vi "HEWH Set Draw Condition.vi"(6 "Station":string, 7 "Condition":T1, 8 "Error In":errorcluster, 9 "Station A Test Sequence":T2[](array[typedef])=[{"Sequence #"=0.0, "Cycles"=0, "Mode Setting"="", "Flow Rate (GPM)"=0.0, "Temperature (F)"=0.0, "Reset Timer"=FALSE, "Use Temp Decline Method"=FALSE, "Terminate Condition"=enum."C1-Terminate Draw @ Gallon Mark", "Condition Value #1"=0.0, "UE"=FALSE, "LE"=FALSE, "Comp"=FALSE, "Fan"=FALSE, "Test End Time (Sec)"=0.0, "Purge Until Cutout"=FALSE, "Start Conditions"=enum."Heat Source Cutout", "Condition Value #2"=0.0, "Remove Power"=FALSE, "Time"=0.0, "Check Special Cond."=enum."SC2-Check Heat Source (On-C2/Off-C1)", "Condition#"=enum."C1", "Draw Flags"=enum."N/A", "Data Processing Delay (FHD 15sec, UEF 5 Sec)"=0.0, "Test Complete"=FALSE, "User Setpoint"=0.0, "Tank Setpoint"=0.0}, {"Sequence #"=0.0, "Cycles"=0, "Mode Setting"="", "Flow Rate (GPM)"=0.0, "Temperature (F)"=0.0, "Reset Timer"=FALSE, "Use Temp Decline Method"=FALSE, "Terminate Condition"=enum."C1-Terminate Draw @ Gallon Mark", "Condition Value #1"=0.0, "UE"=FALSE, "LE"=FALSE, "Comp"=FALSE, "Fan"=FALSE, "Test End Time (Sec)"=0.0, "Purge Until Cutout"=FALSE, "Start Conditions"=enum."Heat Source Cutout", "Condition Value #2"=0.0, "Remove Power"=FALSE, "Time"=0.0, "Check Special Cond."=enum."SC2-Check Heat Source (On-C2/Off-C1)", "Condition#"=enum."C1", "Draw Flags"=enum."N/A", "Data Processing Delay (FHD 15sec, UEF 5 Sec)"=0.0, "Test Complete"=FALSE, "User Setpoint"=0.0, "Tank Setpoint"=0.0}, {"Sequence #"=0.0, "Cycles"=0, "Mode Setting"="", "Flow Rate (GPM)"=0.0, "Temperature (F)"=0.0, "Reset Timer"=FALSE, "Use Temp Decline Method"=FALSE, "Terminate Condition"=enum."C1-Terminate Draw @ Gallon Mark", "Condition Value #1"=0.0, "UE"=FALSE, "LE"=FALSE, "Comp"=FALSE, "Fan"=FALSE, "Test End Time (Sec)"=0.0, "Purge Until Cutout"=FALSE, "Start Conditions"=enum."Heat Source Cutout", "Condition Value #2"=0.0, "Remove Power"=FALSE, "Time"=0.0, "Check Special Cond."=enum."SC2-Check Heat Source (On-C2/Off-C1)", "Condition#"=enum."C1", "Draw Flags"=enum."N/A", "Data Processing Delay (FHD 15sec, UEF 5 Sec)"=0.0, "Test Complete"=FALSE, "User Setpoint"=0.0, "Tank Setpoint"=0.0}, {"Sequence #"=0.0, "Cycles"=0, "Mode Setting"="", "Flow Rate (GPM)"=0.0, "Temperature (F)"=0.0, "Reset Timer"=FALSE, "Use Temp Decline Method"=FALSE, "Terminate Condition"=enum."C1-Terminate Draw @ Gallon Mark", "Condition Value #1"=0.0, "UE"=FALSE, "LE"=FALSE, "Comp"=FALSE, "Fan"=FALSE, "Test End Time (Sec)"=0.0, "Purge Until Cutout"=FALSE, "Start Conditions"=enum."Heat Source Cutout", "Condition Value #2"=0.0, "Remove Power"=FALSE, "Time"=0.0, "Check Special Cond."=enum."SC2-Check Heat Source (On-C2/Off-C1)", "Condition#"=enum."C1", "Draw Flags"=enum."N/A", "Data Processing Delay (FHD 15sec, UEF 5 Sec)"=0.0, "Test Complete"=FALSE, "User Setpoint"=0.0, "Tank Setpoint"=0.0}, {"Sequence #"=0.0, "Cycles"=0, "Mode Setting"="", "Flow Rate (GPM)"=0.0, "Temperature (F)"=0.0, "Reset Timer"=FALSE, "Use Temp Decline Method"=FALSE, "Terminate Condition"=enum."C1-Terminate Draw @ Gallon Mark", "Condition Value #1"=0.0, "UE"=FALSE, "LE"=FALSE, "Comp"=FALSE, "Fan"=FALSE, "Test End Time (Sec)"=0.0, "Purge Until Cutout"=FALSE, "Start Conditions"=enum."Heat Source Cutout", "Condition Value #2"=0.0, "Remove Power"=FALSE, "Time"=0.0, "Check Special Cond."=enum."SC2-Check Heat Source (On-C2/Off-C1)", "Condition#"=enum."C1", "Draw Flags"=enum."N/A", "Data Processing Delay (FHD 15sec, UEF 5 Sec)"=0.0, "Test Complete"=FALSE, "User Setpoint"=0.0, "Tank Setpoint"=0.0}, {"Sequence #"=0.0, "Cycles"=0, "Mode Setting"="", "Flow Rate (GPM)"=0.0, "Temperature (F)"=0.0, "Reset Timer"=FALSE, "Use Temp Decline Method"=FALSE, "Terminate Condition"=enum."C1-Terminate Draw @ Gallon Mark", "Condition Value #1"=0.0, "UE"=FALSE, "LE"=FALSE, "Comp"=FALSE, "Fan"=FALSE, "Test End Time (Sec)"=0.0, "Purge Until Cutout"=FALSE, "Start Conditions"=enum."Heat Source Cutout", "Condition Value #2"=0.0, "Remove Power"=FALSE, "Time"=0.0, "Check Special Cond."=enum."SC2-Check Heat Source (On-C2/Off-C1)", "Condition#"=enum."C1", "Draw Flags"=enum."N/A", "Data Processing Delay (FHD 15sec, UEF 5 Sec)"=0.0, "Test Complete"=FALSE, "User Setpoint"=0.0, "Tank Setpoint"=0.0}, {"Sequence #"=0.0, "Cycles"=0, "Mode Setting"="", "Flow Rate (GPM)"=0.0, "Temperature (F)"=0.0, "Reset Timer"=FALSE, "Use Temp Decline Method"=FALSE, "Terminate Condition"=enum."C1-Terminate Draw @ Gallon Mark", "Condition Value #1"=0.0, "UE"=FALSE, "LE"=FALSE, "Comp"=FALSE, "Fan"=FALSE, "Test End Time (Sec)"=0.0, "Purge Until Cutout"=FALSE, "Start Conditions"=enum."Heat Source Cutout", "Condition Value #2"=0.0, "Remove Power"=FALSE, "Time"=0.0, "Check Special Cond."=enum."SC2-Check Heat Source (On-C2/Off-C1)", "Condition#"=enum."C1", "Draw Flags"=enum."N/A", "Data Processing Delay (FHD 15sec, UEF 5 Sec)"=0.0, "Test Complete"=FALSE, "User Setpoint"=0.0, "Tank Setpoint"=0.0}, {"Sequence #"=0.0, "Cycles"=0, "Mode Setting"="", "Flow Rate (GPM)"=0.0, "Temperature (F)"=0.0, "Reset Timer"=FALSE, "Use Temp Decline Method"=FALSE, "Terminate Condition"=enum."C1-Terminate Draw @ Gallon Mark", "Condition Value #1"=0.0, "UE"=FALSE, "LE"=FALSE, "Comp"=FALSE, "Fan"=FALSE, "Test End Time (Sec)"=0.0, "Purge Until Cutout"=FALSE, "Start Conditions"=enum."Heat Source Cutout", "Condition Value #2"=0.0, "Remove Power"=FALSE, "Time"=0.0, "Check Special Cond."=enum."SC2-Check Heat Source (On-C2/Off-C1)", "Condition#"=enum."C1", "Draw Flags"=enum."N/A", "Data Processing Delay (FHD 15sec, UEF 5 Sec)"=0.0, "Test Complete"=FALSE, "User Setpoint"=0.0, "Tank Setpoint"=0.0}] {"Time" format="%<%H:%M:%S>t"}, 10 "Draw Parameters":T19={"Draws Left"=0, "Draws Left Array"=[], "Remaining Draws (A)"=1000, "Remaining Draws (B)"=1000, "Remaining Draws (C)"=1000, "Remaining Draws (D)"=1000, "Index of Element (A-D)"=[], "Station A"={"Sequence #"=0.0, "Cycles"=0, "Mode Setting"="", "Flow Rate (GPM)"=0.0, "Temperature (F)"=0.0, "Reset Timer"=FALSE, "Use Temp Decline Method"=FALSE, "Terminate Condition"=enum."C1-Terminate Draw @ Gallon Mark", "Condition Value #1"=0.0, "UE"=FALSE, "LE"=FALSE, "Comp"=FALSE, "Fan"=FALSE, "Test End Time (Sec)"=0.0, "Purge Until Cutout"=FALSE, "Start Conditions"=enum."Heat Source Cutout", "Condition Value #2"=0.0, "Remove Power"=FALSE, "Time"=0.0, "Check Special Cond."=enum."SC2-Check Heat Source (On-C2/Off-C1)", "Condition#"=enum."C1", "Draw Flags"=enum."N/A", "Data Processing Delay (FHD 15sec, UEF 5 Sec)"=0.0, "Test Complete"=FALSE, "User Setpoint"=0.0, "Tank Setpoint"=0.0}, "Station B"={"Sequence #"=0.0, "Cycles"=0, "Mode Setting"="", "Flow Rate (GPM)"=0.0, "Temperature (F)"=0.0, "Reset Timer"=FALSE, "Use Temp Decline Method"=FALSE, "Terminate Condition"=enum."C1-Terminate Draw @ Gallon Mark", "Condition Value #1"=0.0, "UE"=FALSE, "LE"=FALSE, "Comp"=FALSE, "Fan"=FALSE, "Test End Time (Sec)"=0.0, "Purge Until Cutout"=FALSE, "Start Conditions"=enum."Heat Source Cutout", "Condition Value #2"=0.0, "Remove Power"=FALSE, "Time"=0.0, "Check Special Cond."=enum."SC2-Check Heat Source (On-C2/Off-C1)", "Condition#"=enum."C1", "Draw Flags"=enum."N/A", "Data Processing Delay (FHD 15sec, UEF 5 Sec)"=0.0, "Test Complete"=FALSE, "User Setpoint"=0.0, "Tank Setpoint"=0.0}, "Station C"={"Sequence #"=0.0, "Cycles"=0, "Mode Setting"="", "Flow Rate (GPM)"=0.0, "Temperature (F)"=0.0, "Reset Timer"=FALSE, "Use Temp Decline Method"=FALSE, "Terminate Condition"=enum."C1-Terminate Draw @ Gallon Mark", "Condition Value #1"=0.0, "UE"=FALSE, "LE"=FALSE, "Comp"=FALSE, "Fan"=FALSE, "Test End Time (Sec)"=0.0, "Purge Until Cutout"=FALSE, "Start Conditions"=enum."Heat Source Cutout", "Condition Value #2"=0.0, "Remove Power"=FALSE, "Time"=0.0, "Check Special Cond."=enum."SC2-Check Heat Source (On-C2/Off-C1)", "Condition#"=enum."C1", "Draw Flags"=enum."N/A", "Data Processing Delay (FHD 15sec, UEF 5 Sec)"=0.0, "Test Complete"=FALSE, "User Setpoint"=0.0, "Tank Setpoint"=0.0}, "Station D"={"Sequence #"=0.0, "Cycles"=0, "Mode Setting"="", "Flow Rate (GPM)"=0.0, "Temperature (F)"=0.0, "Reset Timer"=FALSE, "Use Temp Decline Method"=FALSE, "Terminate Condition"=enum."C1-Terminate Draw @ Gallon Mark", "Condition Value #1"=0.0, "UE"=FALSE, "LE"=FALSE, "Comp"=FALSE, "Fan"=FALSE, "Test End Time (Sec)"=0.0, "Purge Until Cutout"=FALSE, "Start Conditions"=enum."Heat Source Cutout", "Condition Value #2"=0.0, "Remove Power"=FALSE, "Time"=0.0, "Check Special Cond."=enum."SC2-Check Heat Source (On-C2/Off-C1)", "Condition#"=enum."C1", "Draw Flags"=enum."N/A", "Data Processing Delay (FHD 15sec, UEF 5 Sec)"=0.0, "Test Complete"=FALSE, "User Setpoint"=0.0, "Tank Setpoint"=0.0}} {"Station D"."Time" format="%<%H:%M:%S>t"; "Station C"."Time" format="%<%H:%M:%S>t"; "Station B"."Time" format="%<%H:%M:%S>t"; "Station A"."Time" format="%<%H:%M:%S>t"}, 11 "Core HEWH Data Input":T8={"Scan Rate Adjust"=0.0, "Draw Count"=0, "Test Patten Setup"={"Total Gallons Schedule"=[], "PRAT/RLT Sequence"=[{"Sequence #"=1.0, "Cycles"=35, "Mode Setting"="", "Flow Rate (GPM)"=0.0, "Temperature (F)"=0.0, "Reset Timer"=FALSE, "Use Temp Decline Method"=FALSE, "Terminate Condition"=enum."C1-Terminate Draw @ Gallon Mark", "Condition Value #1"=0.0, "UE"=FALSE, "LE"=FALSE, "Comp"=FALSE, "Fan"=FALSE, "Test End Time (Sec)"=0.0, "Purge Until Cutout"=FALSE, "Start Conditions"=enum."Heat Source Cutout", "Condition Value #2"=0.0, "Remove Power"=FALSE, "Time"=0.0, "Check Special Cond."=enum."SC2-Check Heat Source (On-C2/Off-C1)", "Condition#"=enum."C1", "Draw Flags"=enum."N/A", "Data Processing Delay (FHD 15sec, UEF 5 Sec)"=0.0, "Test Complete"=FALSE, "User Setpoint"=0.0, "Tank Setpoint"=0.0}, {"Sequence #"=2.0, "Cycles"=15, "Mode Setting"="", "Flow Rate (GPM)"=0.0, "Temperature (F)"=0.0, "Reset Timer"=FALSE, "Use Temp Decline Method"=FALSE, "Terminate Condition"=enum."C1-Terminate Draw @ Gallon Mark", "Condition Value #1"=0.0, "UE"=FALSE, "LE"=FALSE, "Comp"=FALSE, "Fan"=FALSE, "Test End Time (Sec)"=0.0, "Purge Until Cutout"=FALSE, "Start Conditions"=enum."Heat Source Cutout", "Condition Value #2"=0.0, "Remove Power"=FALSE, "Time"=0.0, "Check Special Cond."=enum."SC2-Check Heat Source (On-C2/Off-C1)", "Condition#"=enum."C1", "Draw Flags"=enum."N/A", "Data Processing Delay (FHD 15sec, UEF 5 Sec)"=0.0, "Test Complete"=FALSE, "User Setpoint"=0.0, "Tank Setpoint"=0.0}, {"Sequence #"=3.0, "Cycles"=35, "Mode Setting"="", "Flow Rate (GPM)"=0.0, "Temperature (F)"=0.0, "Reset Timer"=FALSE, "Use Temp Decline Method"=FALSE, "Terminate Condition"=enum."C1-Terminate Draw @ Gallon Mark", "Condition Value #1"=0.0, "UE"=FALSE, "LE"=FALSE, "Comp"=FALSE, "Fan"=FALSE, "Test End Time (Sec)"=0.0, "Purge Until Cutout"=FALSE, "Start Conditions"=enum."Heat Source Cutout", "Condition Value #2"=0.0, "Remove Power"=FALSE, "Time"=0.0, "Check Special Cond."=enum."SC2-Check Heat Source (On-C2/Off-C1)", "Condition#"=enum."C1", "Draw Flags"=enum."N/A", "Data Processing Delay (FHD 15sec, UEF 5 Sec)"=0.0, "Test Complete"=FALSE, "User Setpoint"=0.0, "Tank Setpoint"=0.0}, {"Sequence #"=4.0, "Cycles"=15, "Mode Setting"="", "Flow Rate (GPM)"=0.0, "Temperature (F)"=0.0, "Reset Timer"=FALSE, "Use Temp Decline Method"=FALSE, "Terminate Condition"=enum."C1-Terminate Draw @ Gallon Mark", "Condition Value #1"=0.0, "UE"=FALSE, "LE"=FALSE, "Comp"=FALSE, "Fan"=FALSE, "Test End Time (Sec)"=0.0, "Purge Until Cutout"=FALSE, "Start Conditions"=enum."Heat Source Cutout", "Condition Value #2"=0.0, "Remove Power"=FALSE, "Time"=0.0, "Check Special Cond."=enum."SC2-Check Heat Source (On-C2/Off-C1)", "Condition#"=enum."C1", "Draw Flags"=enum."N/A", "Data Processing Delay (FHD 15sec, UEF 5 Sec)"=0.0, "Test Complete"=FALSE, "User Setpoint"=0.0, "Tank Setpoint"=0.0}, {"Sequence #"=5.0, "Cycles"=35, "Mode Setting"="", "Flow Rate (GPM)"=0.0, "Temperature (F)"=0.0, "Reset Timer"=FALSE, "Use Temp Decline Method"=FALSE, "Terminate Condition"=enum."C1-Terminate Draw @ Gallon Mark", "Condition Value #1"=0.0, "UE"=FALSE, "LE"=FALSE, "Comp"=FALSE, "Fan"=FALSE, "Test End Time (Sec)"=0.0, "Purge Until Cutout"=FALSE, "Start Conditions"=enum."Heat Source Cutout", "Condition Value #2"=0.0, "Remove Power"=FALSE, "Time"=0.0, "Check Special Cond."=enum."SC2-Check Heat Source (On-C2/Off-C1)", "Condition#"=enum."C1", "Draw Flags"=enum."N/A", "Data Processing Delay (FHD 15sec, UEF 5 Sec)"=0.0, "Test Complete"=FALSE, "User Setpoint"=0.0, "Tank Setpoint"=0.0}, {"Sequence #"=6.0, "Cycles"=15, "Mode Setting"="", "Flow Rate (GPM)"=0.0, "Temperature (F)"=0.0, "Reset Timer"=FALSE, "Use Temp Decline Method"=FALSE, "Terminate Condition"=enum."C1-Terminate Draw @ Gallon Mark", "Condition Value #1"=0.0, "UE"=FALSE, "LE"=FALSE, "Comp"=FALSE, "Fan"=FALSE, "Test End Time (Sec)"=0.0, "Purge Until Cutout"=FALSE, "Start Conditions"=enum."Heat Source Cutout", "Condition Value #2"=0.0, "Remove Power"=FALSE, "Time"=0.0, "Check Special Cond."=enum."SC2-Check Heat Source (On-C2/Off-C1)", "Condition#"=enum."C1", "Draw Flags"=enum."N/A", "Data Processing Delay (FHD 15sec, UEF 5 Sec)"=0.0, "Test Complete"=FALSE, "User Setpoint"=0.0, "Tank Setpoint"=0.0}, {"Sequence #"=7.0, "Cycles"=35, "Mode Setting"="", "Flow Rate (GPM)"=0.0, "Temperature (F)"=0.0, "Reset Timer"=FALSE, "Use Temp Decline Method"=FALSE, "Terminate Condition"=enum."C1-Terminate Draw @ Gallon Mark", "Condition Value #1"=0.0, "UE"=FALSE, "LE"=FALSE, "Comp"=FALSE, "Fan"=FALSE, "Test End Time (Sec)"=0.0, "Purge Until Cutout"=FALSE, "Start Conditions"=enum."Heat Source Cutout", "Condition Value #2"=0.0, "Remove Power"=FALSE, "Time"=0.0, "Check Special Cond."=enum."SC2-Check Heat Source (On-C2/Off-C1)", "Condition#"=enum."C1", "Draw Flags"=enum."N/A", "Data Processing Delay (FHD 15sec, UEF 5 Sec)"=0.0, "Test Complete"=FALSE, "User Setpoint"=0.0, "Tank Setpoint"=0.0}, {"Sequence #"=8.0, "Cycles"=15, "Mode Setting"="", "Flow Rate (GPM)"=0.0, "Temperature (F)"=0.0, "Reset Timer"=FALSE, "Use Temp Decline Method"=FALSE, "Terminate Condition"=enum."C1-Terminate Draw @ Gallon Mark", "Condition Value #1"=0.0, "UE"=FALSE, "LE"=FALSE, "Comp"=FALSE, "Fan"=FALSE, "Test End Time (Sec)"=0.0, "Purge Until Cutout"=FALSE, "Start Conditions"=enum."Heat Source Cutout", "Condition Value #2"=0.0, "Remove Power"=FALSE, "Time"=0.0, "Check Special Cond."=enum."SC2-Check Heat Source (On-C2/Off-C1)", "Condition#"=enum."C1", "Draw Flags"=enum."N/A", "Data Processing Delay (FHD 15sec, UEF 5 Sec)"=0.0, "Test Complete"=FALSE, "User Setpoint"=0.0, "Tank Setpoint"=0.0}], "Current Sequence Index"=0}, "HEWH Specific DAQ"={"HEWH Data"={"HEWH Standard"={"Voltage (Volts)"=0.0, "Current (Amps)"=0.0, "Power (Watts)"=0.0, "WattHours (Wh)"=0.0, "TC Tree (AVG)"=0.0, "Flow Rate (GPM)"=0.0, "Gallons (Gal)"=0.0, "RTD Out (Deg F)"=0.0, "RTD In (Deg F)"=0.0, "RTD Amb (Deg F)"=0.0, "TC Down"=0.0, "UE Event Lead"=0, "LE Event Lead"=0, "TC Tree Array"=[]}, "PRAT"={"Power (Watts) A"=0.0, "Power (Watts) B"=0.0, "Power (Watts) C"=0.0, "Power (Watts) D"=0.0, "TC1"=0.0, "TC2"=0.0, "TC3"=0.0, "TC4"=0.0, "WattHours (Wh) A"=0.0, "WattHours (Wh) B"=0.0, "WattHours (Wh) C"=0.0, "WattHours (Wh) D"=0.0, "Ambient"=0.0, "Extra Temp"=0.0}, "Additional Power Data"={"Vthd"=0.0, "Frequency (Hz)"=0.0, "Apparent Power (VA)"=0.0, "Power Factor"=0.0, "Current Crest Factor"=0.0, "Voltage Crest Factor"=0.0, "Integration Time (sec)"=0.0}}, "Flow Valve % Open"=0.0, "Power State"={"UE"=FALSE, "LE"=FALSE, "COMP"=FALSE, "FANS"=FALSE}, "Power Analyzer"=enum."", "Flow Valve uA Output"=0, "Gallons Start (Gal)"=0.0}, "Test Output Data"={"PreDraw Data Table"=[], "Data Table"=[], "MW100 TC Headers"=[]}, "Calc and Calibration"={"Mean SD Var Max Min Array"=[], "Draw Statistics (DBL)"=[], "Calibration Coefficients DBL"=[], "Start Gallons"=0.0, "Starting Temp Decline"=0.0, "K-Factor (Temperature)"=100.0, "All Draw Stats"=[], "RTD Terminate Value"=0.0, "K-Factor (Flow)"=0.0, "Intellifaucet Type"="", "Gas Thermal Stabilization Array"=[], "Gas Thermal Stabil Complete"=FALSE, "Gas Thermal Time"=0.0, "Therm Reset Cmpt 1"=FALSE, "Therm Reset Cmpt 2"=FALSE, "Last Flow Rate (Therm)"=0.0, "State"=enum."State 1", "Gas Thermal Time 2"=0.0}, "Current Draw Time"=0.0, "LV Program"=enum."HEWH", "Station ID"=enum."A", "Current Cond"=enum."N/A", "Test Complete"=FALSE, "ANSI Rate"={"Array 1"=[], "Array 3"=[], "Array 2"=[], "Start ANSI"=FALSE, "ANSI Start Time"=0.0, "Restart ANSI"=FALSE, "15 Min ANSI Avg (BTU/hr)"=0.0, "20 Min ANSI Avg (BTU/hr)"=0.0, "25 Min ANSI Avg (BTU/hr)"=0.0, "Absolute Pressure"=0.0, "Gas Temperature"=0.0, "Volumetric Flow Rate"=0.0, "Mass Flow Rate"=0.0, "Array 4"=[], "Array 5"=[], "Gas Rate"=0.0, "15 Min Pres Avg (PSIA)"=0.0, "20 Min Pres Avg (PSIA)"=0.0, "25 Min Pres Avg (PSIA)"=0.0, "15 Min Temp Avg (°F) "=0.0, "20 Min Temp Avg (°F)"=0.0, "25 Min Temp Avg (°F)"=0.0, "15 Min Uncorrected Avg (CFH)"=0.0, "20 Min Uncorrected Avg (CFH)"=0.0, "25 Min Uncorrected Avg (CFH)"=0.0, "15 Min Corrected Avg (SCFH)"=0.0, "20 Min Corrected Avg (SCFH)"=0.0, "25 Min Corrected Avg (SCFH)"=0.0, "15 Min Complete"=FALSE, "20 Min Complete"=FALSE, "25 Min Complete"=FALSE, "Heating Value (BTU/ft³)"=0.0}, "Gas Measurment Data"={"Absolute Pressure"=0.0, "Gauge/Diff. Pressure"=0.0, "Barometric Pressure"=0.0, "Temperature"=0.0, "Volumetric Flow"=0.0, "Mass Flow"=0.0, "Setpoint"=0.0, "Valve Drive"=0.0, "Totalizer"=0.0, "[hr]"=0.0, "[min]"=0.0, "[sec]"=0.0, "Totalizer Average Flow"=0.0, "Totalizer Peak Flow"=0.0, "Gas selected"=""}} {"Test Patten Setup"."PRAT/RLT Sequence"."Time" format="%<%H:%M:%S>t"; "Test Patten Setup"."Total Gallons Schedule" format="%.2f"}) -> (0 "Error Out":errorcluster, 3 "Core HEWH Data Output":T8={"Scan Rate Adjust"=0.0, "Draw Count"=0, "Test Patten Setup"={"Total Gallons Schedule"=[], "PRAT/RLT Sequence"=[{"Sequence #"=1.0, "Cycles"=35, "Mode Setting"="", "Flow Rate (GPM)"=0.0, "Temperature (F)"=0.0, "Reset Timer"=FALSE, "Use Temp Decline Method"=FALSE, "Terminate Condition"=enum."C1-Terminate Draw @ Gallon Mark", "Condition Value #1"=0.0, "UE"=FALSE, "LE"=FALSE, "Comp"=FALSE, "Fan"=FALSE, "Test End Time (Sec)"=0.0, "Purge Until Cutout"=FALSE, "Start Conditions"=enum."Heat Source Cutout", "Condition Value #2"=0.0, "Remove Power"=FALSE, "Time"=0.0, "Check Special Cond."=enum."SC2-Check Heat Source (On-C2/Off-C1)", "Condition#"=enum."C1", "Draw Flags"=enum."N/A", "Data Processing Delay (FHD 15sec, UEF 5 Sec)"=0.0, "Test Complete"=FALSE, "User Setpoint"=0.0, "Tank Setpoint"=0.0}, {"Sequence #"=2.0, "Cycles"=15, "Mode Setting"="", "Flow Rate (GPM)"=0.0, "Temperature (F)"=0.0, "Reset Timer"=FALSE, "Use Temp Decline Method"=FALSE, "Terminate Condition"=enum."C1-Terminate Draw @ Gallon Mark", "Condition Value #1"=0.0, "UE"=FALSE, "LE"=FALSE, "Comp"=FALSE, "Fan"=FALSE, "Test End Time (Sec)"=0.0, "Purge Until Cutout"=FALSE, "Start Conditions"=enum."Heat Source Cutout", "Condition Value #2"=0.0, "Remove Power"=FALSE, "Time"=0.0, "Check Special Cond."=enum."SC2-Check Heat Source (On-C2/Off-C1)", "Condition#"=enum."C1", "Draw Flags"=enum."N/A", "Data Processing Delay (FHD 15sec, UEF 5 Sec)"=0.0, "Test Complete"=FALSE, "User Setpoint"=0.0, "Tank Setpoint"=0.0}, {"Sequence #"=3.0, "Cycles"=35, "Mode Setting"="", "Flow Rate (GPM)"=0.0, "Temperature (F)"=0.0, "Reset Timer"=FALSE, "Use Temp Decline Method"=FALSE, "Terminate Condition"=enum."C1-Terminate Draw @ Gallon Mark", "Condition Value #1"=0.0, "UE"=FALSE, "LE"=FALSE, "Comp"=FALSE, "Fan"=FALSE, "Test End Time (Sec)"=0.0, "Purge Until Cutout"=FALSE, "Start Conditions"=enum."Heat Source Cutout", "Condition Value #2"=0.0, "Remove Power"=FALSE, "Time"=0.0, "Check Special Cond."=enum."SC2-Check Heat Source (On-C2/Off-C1)", "Condition#"=enum."C1", "Draw Flags"=enum."N/A", "Data Processing Delay (FHD 15sec, UEF 5 Sec)"=0.0, "Test Complete"=FALSE, "User Setpoint"=0.0, "Tank Setpoint"=0.0}, {"Sequence #"=4.0, "Cycles"=15, "Mode Setting"="", "Flow Rate (GPM)"=0.0, "Temperature (F)"=0.0, "Reset Timer"=FALSE, "Use Temp Decline Method"=FALSE, "Terminate Condition"=enum."C1-Terminate Draw @ Gallon Mark", "Condition Value #1"=0.0, "UE"=FALSE, "LE"=FALSE, "Comp"=FALSE, "Fan"=FALSE, "Test End Time (Sec)"=0.0, "Purge Until Cutout"=FALSE, "Start Conditions"=enum."Heat Source Cutout", "Condition Value #2"=0.0, "Remove Power"=FALSE, "Time"=0.0, "Check Special Cond."=enum."SC2-Check Heat Source (On-C2/Off-C1)", "Condition#"=enum."C1", "Draw Flags"=enum."N/A", "Data Processing Delay (FHD 15sec, UEF 5 Sec)"=0.0, "Test Complete"=FALSE, "User Setpoint"=0.0, "Tank Setpoint"=0.0}, {"Sequence #"=5.0, "Cycles"=35, "Mode Setting"="", "Flow Rate (GPM)"=0.0, "Temperature (F)"=0.0, "Reset Timer"=FALSE, "Use Temp Decline Method"=FALSE, "Terminate Condition"=enum."C1-Terminate Draw @ Gallon Mark", "Condition Value #1"=0.0, "UE"=FALSE, "LE"=FALSE, "Comp"=FALSE, "Fan"=FALSE, "Test End Time (Sec)"=0.0, "Purge Until Cutout"=FALSE, "Start Conditions"=enum."Heat Source Cutout", "Condition Value #2"=0.0, "Remove Power"=FALSE, "Time"=0.0, "Check Special Cond."=enum."SC2-Check Heat Source (On-C2/Off-C1)", "Condition#"=enum."C1", "Draw Flags"=enum."N/A", "Data Processing Delay (FHD 15sec, UEF 5 Sec)"=0.0, "Test Complete"=FALSE, "User Setpoint"=0.0, "Tank Setpoint"=0.0}, {"Sequence #"=6.0, "Cycles"=15, "Mode Setting"="", "Flow Rate (GPM)"=0.0, "Temperature (F)"=0.0, "Reset Timer"=FALSE, "Use Temp Decline Method"=FALSE, "Terminate Condition"=enum."C1-Terminate Draw @ Gallon Mark", "Condition Value #1"=0.0, "UE"=FALSE, "LE"=FALSE, "Comp"=FALSE, "Fan"=FALSE, "Test End Time (Sec)"=0.0, "Purge Until Cutout"=FALSE, "Start Conditions"=enum."Heat Source Cutout", "Condition Value #2"=0.0, "Remove Power"=FALSE, "Time"=0.0, "Check Special Cond."=enum."SC2-Check Heat Source (On-C2/Off-C1)", "Condition#"=enum."C1", "Draw Flags"=enum."N/A", "Data Processing Delay (FHD 15sec, UEF 5 Sec)"=0.0, "Test Complete"=FALSE, "User Setpoint"=0.0, "Tank Setpoint"=0.0}, {"Sequence #"=7.0, "Cycles"=35, "Mode Setting"="", "Flow Rate (GPM)"=0.0, "Temperature (F)"=0.0, "Reset Timer"=FALSE, "Use Temp Decline Method"=FALSE, "Terminate Condition"=enum."C1-Terminate Draw @ Gallon Mark", "Condition Value #1"=0.0, "UE"=FALSE, "LE"=FALSE, "Comp"=FALSE, "Fan"=FALSE, "Test End Time (Sec)"=0.0, "Purge Until Cutout"=FALSE, "Start Conditions"=enum."Heat Source Cutout", "Condition Value #2"=0.0, "Remove Power"=FALSE, "Time"=0.0, "Check Special Cond."=enum."SC2-Check Heat Source (On-C2/Off-C1)", "Condition#"=enum."C1", "Draw Flags"=enum."N/A", "Data Processing Delay (FHD 15sec, UEF 5 Sec)"=0.0, "Test Complete"=FALSE, "User Setpoint"=0.0, "Tank Setpoint"=0.0}, {"Sequence #"=8.0, "Cycles"=15, "Mode Setting"="", "Flow Rate (GPM)"=0.0, "Temperature (F)"=0.0, "Reset Timer"=FALSE, "Use Temp Decline Method"=FALSE, "Terminate Condition"=enum."C1-Terminate Draw @ Gallon Mark", "Condition Value #1"=0.0, "UE"=FALSE, "LE"=FALSE, "Comp"=FALSE, "Fan"=FALSE, "Test End Time (Sec)"=0.0, "Purge Until Cutout"=FALSE, "Start Conditions"=enum."Heat Source Cutout", "Condition Value #2"=0.0, "Remove Power"=FALSE, "Time"=0.0, "Check Special Cond."=enum."SC2-Check Heat Source (On-C2/Off-C1)", "Condition#"=enum."C1", "Draw Flags"=enum."N/A", "Data Processing Delay (FHD 15sec, UEF 5 Sec)"=0.0, "Test Complete"=FALSE, "User Setpoint"=0.0, "Tank Setpoint"=0.0}], "Current Sequence Index"=0}, "HEWH Specific DAQ"={"HEWH Data"={"HEWH Standard"={"Voltage (Volts)"=0.0, "Current (Amps)"=0.0, "Power (Watts)"=0.0, "WattHours (Wh)"=0.0, "TC Tree (AVG)"=0.0, "Flow Rate (GPM)"=0.0, "Gallons (Gal)"=0.0, "RTD Out (Deg F)"=0.0, "RTD In (Deg F)"=0.0, "RTD Amb (Deg F)"=0.0, "TC Down"=0.0, "UE Event Lead"=0, "LE Event Lead"=0, "TC Tree Array"=[]}, "PRAT"={"Power (Watts) A"=0.0, "Power (Watts) B"=0.0, "Power (Watts) C"=0.0, "Power (Watts) D"=0.0, "TC1"=0.0, "TC2"=0.0, "TC3"=0.0, "TC4"=0.0, "WattHours (Wh) A"=0.0, "WattHours (Wh) B"=0.0, "WattHours (Wh) C"=0.0, "WattHours (Wh) D"=0.0, "Ambient"=0.0, "Extra Temp"=0.0}, "Additional Power Data"={"Vthd"=0.0, "Frequency (Hz)"=0.0, "Apparent Power (VA)"=0.0, "Power Factor"=0.0, "Current Crest Factor"=0.0, "Voltage Crest Factor"=0.0, "Integration Time (sec)"=0.0}}, "Flow Valve % Open"=0.0, "Power State"={"UE"=FALSE, "LE"=FALSE, "COMP"=FALSE, "FANS"=FALSE}, "Power Analyzer"=enum."", "Flow Valve uA Output"=0, "Gallons Start (Gal)"=0.0}, "Test Output Data"={"PreDraw Data Table"=[], "Data Table"=[], "MW100 TC Headers"=[]}, "Calc and Calibration"={"Mean SD Var Max Min Array"=[], "Draw Statistics (DBL)"=[], "Calibration Coefficients DBL"=[], "Start Gallons"=0.0, "Starting Temp Decline"=0.0, "K-Factor (Temperature)"=100.0, "All Draw Stats"=[], "RTD Terminate Value"=0.0, "K-Factor (Flow)"=0.0, "Intellifaucet Type"="", "Gas Thermal Stabilization Array"=[], "Gas Thermal Stabil Complete"=FALSE, "Gas Thermal Time"=0.0, "Therm Reset Cmpt 1"=FALSE, "Therm Reset Cmpt 2"=FALSE, "Last Flow Rate (Therm)"=0.0, "State"=enum."State 1", "Gas Thermal Time 2"=0.0}, "Current Draw Time"=0.0, "LV Program"=enum."HEWH", "Station ID"=enum."A", "Current Cond"=enum."N/A", "Test Complete"=FALSE, "ANSI Rate"={"Array 1"=[], "Array 3"=[], "Array 2"=[], "Start ANSI"=FALSE, "ANSI Start Time"=0.0, "Restart ANSI"=FALSE, "15 Min ANSI Avg (BTU/hr)"=0.0, "20 Min ANSI Avg (BTU/hr)"=0.0, "25 Min ANSI Avg (BTU/hr)"=0.0, "Absolute Pressure"=0.0, "Gas Temperature"=0.0, "Volumetric Flow Rate"=0.0, "Mass Flow Rate"=0.0, "Array 4"=[], "Array 5"=[], "Gas Rate"=0.0, "15 Min Pres Avg (PSIA)"=0.0, "20 Min Pres Avg (PSIA)"=0.0, "25 Min Pres Avg (PSIA)"=0.0, "15 Min Temp Avg (°F) "=0.0, "20 Min Temp Avg (°F)"=0.0, "25 Min Temp Avg (°F)"=0.0, "15 Min Uncorrected Avg (CFH)"=0.0, "20 Min Uncorrected Avg (CFH)"=0.0, "25 Min Uncorrected Avg (CFH)"=0.0, "15 Min Corrected Avg (SCFH)"=0.0, "20 Min Corrected Avg (SCFH)"=0.0, "25 Min Corrected Avg (SCFH)"=0.0, "15 Min Complete"=FALSE, "20 Min Complete"=FALSE, "25 Min Complete"=FALSE, "Heating Value (BTU/ft³)"=0.0}, "Gas Measurment Data"={"Absolute Pressure"=0.0, "Gauge/Diff. Pressure"=0.0, "Barometric Pressure"=0.0, "Temperature"=0.0, "Volumetric Flow"=0.0, "Mass Flow"=0.0, "Setpoint"=0.0, "Valve Drive"=0.0, "Totalizer"=0.0, "[hr]"=0.0, "[min]"=0.0, "[sec]"=0.0, "Totalizer Average Flow"=0.0, "Totalizer Peak Flow"=0.0, "Gas selected"=""}} {"Test Patten Setup"."PRAT/RLT Sequence"."Time" format="%<%H:%M:%S>t"; "Test Patten Setup"."Total Gallons Schedule" format="%.2f"})   [LabVIEW 2019]
uses:
  Type Definitions/HEWH Draw Parameters.ctl
  Type Definitions/PRAT Test.ctl
  Utility/Save File/File Setup (Public)/Type Definition/Save File HEWH Heating Control Mode.ctl
  Type Definitions/Terminate Draw Conditions.ctl
  Type Definitions/HEWH Start Conditions.ctl
  Type Definitions/Check Special Condtions.ctl
  Type Definitions/HEWH Special Condition Check.ctl
  Type Definitions/HEWH Draw Flag ENUM.ctl
  Type Definitions/HEWH Output Information.ctl
  Type Definitions/HEWH Draw Pattern Setup.ctl
  Type Definitions/HEWH Specific DAQ.ctl
  Type Definitions/HEWH Power Data.ctl
  Type Definitions/HEWH Power Elements.ctl
  Utility/Type Definitions/UTILITY Power Analyzer.ctl
  Type Definitions/HEWH Calc and Calibration.ctl
  Utility/Save File/File Setup (Public)/Type Definition/Save File DOE LabView Program.ctl
  Custom Instrument Control/MW100/Type Definitions/Station ID Selector.ctl
  Range/Type Definitions/RANGE ANSI Rate.ctl
  Drivers/Alicat Gas Meter Driver/Sub-VIs/Data Cluster.ctl
  Utility/Save File/File Setup.lvlib
panel:
  # "Totalizer Timer"
  # "Draw Pattern Setup (24 Hour)"
  # "Totalizer Timer"
  # "Draw Pattern Setup (24 Hour)"
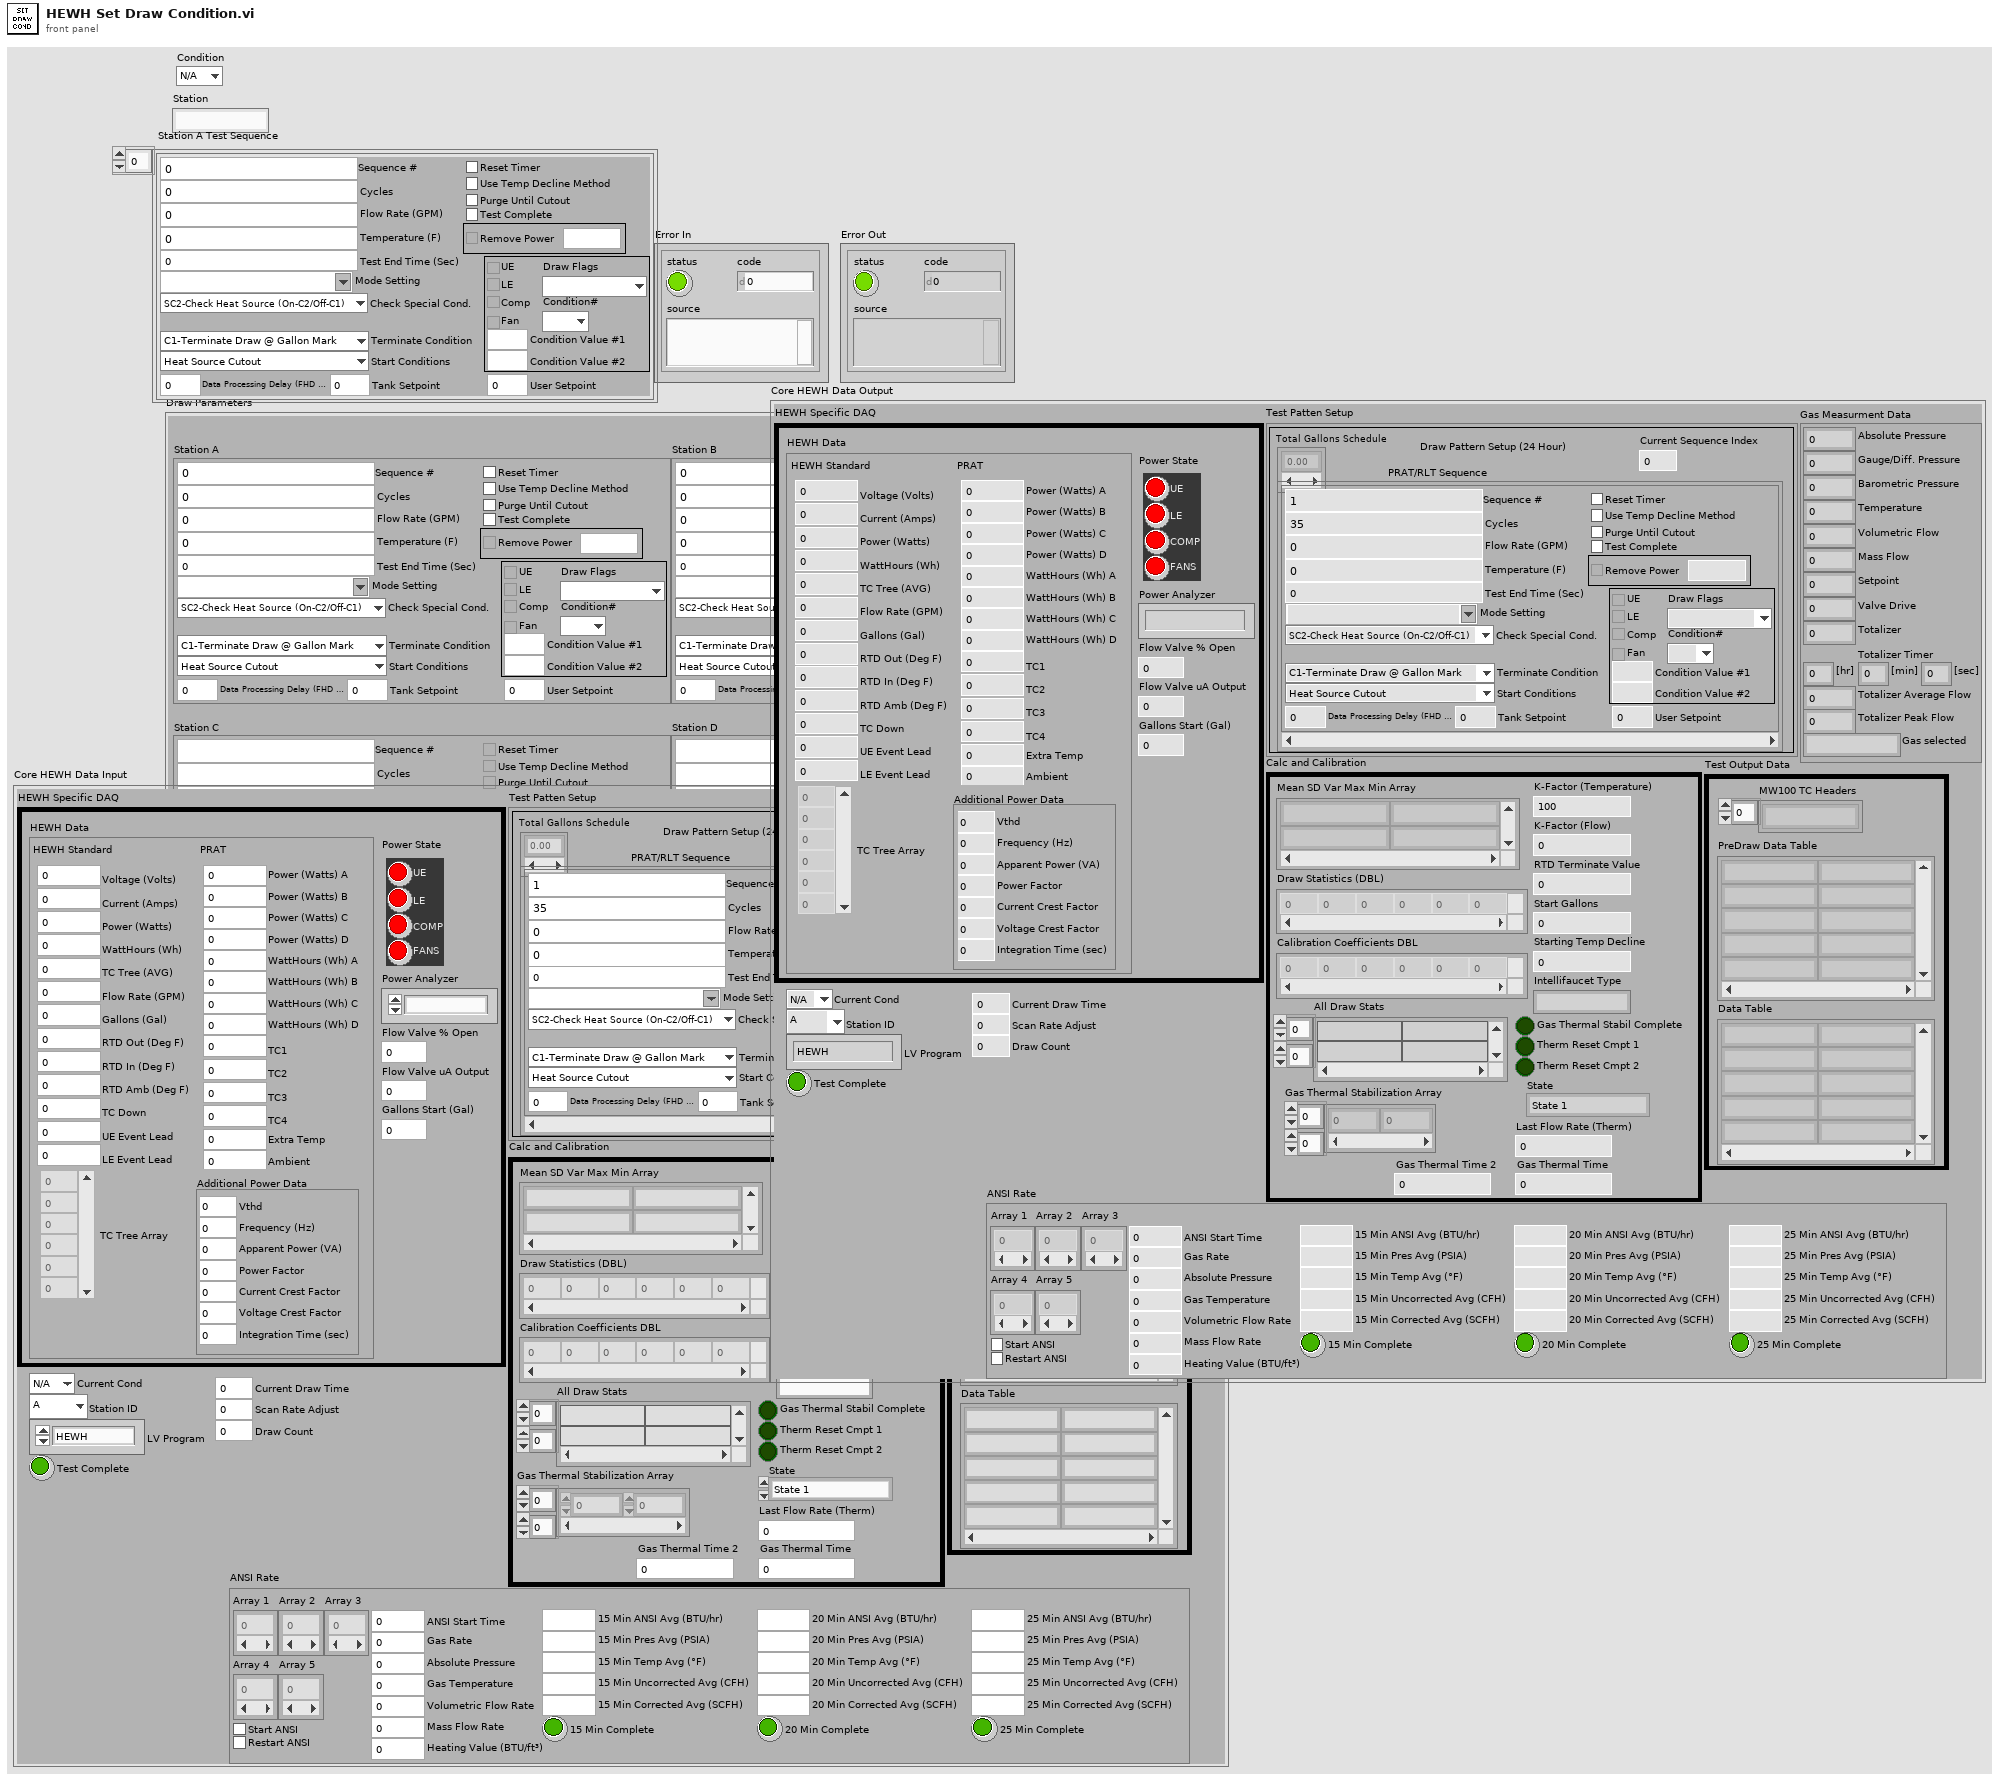
[diagram p1: front panel]
types:
  T1 = typedef "HEWH Special Condition Check.ctl" = enum16{"N/A", "C1", "C2", "Reset/Fail", "Skip Draw Sequence"}
  T2 = typedef "PRAT Test.ctl" = cluster{"Sequence #":dbl, "Cycles":i32, "Mode Setting":T3, "Flow Rate (GPM)":dbl, "Temperature (F)":dbl, "Reset Timer":bool, "Use Temp Decline Method":bool, "Terminate Condition":T4, "Condition Value #1":dbl, "UE":bool, "LE":bool, "Comp":bool, "Fan":bool, "Test End Time (Sec)":dbl, "Purge Until Cutout":bool, "Start Conditions":T5, "Condition Value #2":dbl, "Remove Power":bool, "Time":dbl, "Check Special Cond.":T6, "Condition#":T1, "Draw Flags":T7, "Data Processing Delay (FHD 15sec, UEF 5 Sec)":dbl, "Test Complete":bool, "User Setpoint":dbl, "Tank Setpoint":dbl}
  T3 = typedef "File Setup.lvlib/Save File HEWH Heating Control Mode.ctl" = string
  T4 = typedef "Terminate Draw Conditions.ctl" = enum16{"C1-Terminate Draw @ Gallon Mark", "C2-Special Last Draw (HU Test)", "C3-RTD Out <=", "C4-Mean Tank Temp <=", "C5-Decrease RTD Out (Deg F)", "C6-Time (Seconds)", "C7-Until Any Heat Source", "C8-Specific Heat Source", "C9-Do Nothing", "C10-Inlet Outlet RTD Temp Delta"}
  T5 = typedef "HEWH Start Conditions.ctl" = enum16{"Heat Source Cutout", "At Time (Seconds)", "Every X (Seconds)", "T2 >= X° Below Setpoint", "Seconds From Complete", "Wait for LE & Comp Cutout", "Wait for Comp Cutout", "Wait for LE Cutout", "Wait for UE Cutout", "Start Immediately"}
  T6 = typedef "Check Special Condtions.ctl" = enum16{"SC1-Do Nothing", "SC2-Check Heat Source (On-C2/Off-C1)", "SC3-Check Skip Condition", "SC4-Check Heat Source ON/Fail", "SC5-Keep Draw Valves Open", "SC6-Skip Purge"}
  T7 = typedef "HEWH Draw Flag ENUM.ctl" = enum16{"N/A", "None(0)", "Sml(1)", "Med(2)", "SmlMed(3)", "Lrg(4)", "SmlLrg(5)", "MedLrg(6)", "SmlMedLrg(7)"}
  T8 = typedef "HEWH Output Information.ctl" = cluster{"Scan Rate Adjust":dbl, "Draw Count":i32, "Test Patten Setup":T9, "HEWH Specific DAQ":T10, "Test Output Data":cluster{"PreDraw Data Table":string[][], "Data Table":string[][], "MW100 TC Headers":string[]}, "Calc and Calibration":T14, "Current Draw Time":dbl, "LV Program":T15, "Station ID":T16, "Current Cond":T1, "Test Complete":bool, "ANSI Rate":T17, "Gas Measurment Data":T18}
  T9 = typedef "HEWH Draw Pattern Setup.ctl" = cluster{"Total Gallons Schedule":dbl[], "PRAT/RLT Sequence":T2[], "Current Sequence Index":i32}
  T10 = typedef "HEWH Specific DAQ.ctl" = cluster{"HEWH Data":T11, "Flow Valve % Open":dbl, "Power State":T12, "Power Analyzer":T13, "Flow Valve uA Output":i32, "Gallons Start (Gal)":dbl}
  T11 = typedef "HEWH Power Data.ctl" = cluster{"HEWH Standard":cluster{"Voltage (Volts)":dbl, "Current (Amps)":dbl, "Power (Watts)":dbl, "WattHours (Wh)":dbl, "TC Tree (AVG)":dbl, "Flow Rate (GPM)":dbl, "Gallons (Gal)":dbl, "RTD Out (Deg F)":dbl, "RTD In (Deg F)":dbl, "RTD Amb (Deg F)":dbl, "TC Down":dbl, "UE Event Lead":i32, "LE Event Lead":i32, "TC Tree Array":dbl[]}, "PRAT":cluster{"Power (Watts) A":dbl, "Power (Watts) B":dbl, "Power (Watts) C":dbl, "Power (Watts) D":dbl, "TC1":dbl, "TC2":dbl, "TC3":dbl, "TC4":dbl, "WattHours (Wh) A":dbl, "WattHours (Wh) B":dbl, "WattHours (Wh) C":dbl, "WattHours (Wh) D":dbl, "Ambient":dbl, "Extra Temp":dbl}, "Additional Power Data":cluster{"Vthd":dbl, "Frequency (Hz)":dbl, "Apparent Power (VA)":dbl, "Power Factor":dbl, "Current Crest Factor":dbl, "Voltage Crest Factor":dbl, "Integration Time (sec)":dbl}}
  T12 = typedef "HEWH Power Elements.ctl" = cluster{"UE":bool, "LE":bool, "COMP":bool, "FANS":bool}
  T13 = typedef "UTILITY Power Analyzer.ctl" = enum16{"", "APLUS", "WT210", "WT500", "WT300", "OSI", "Debug", "WT230", "WT300_1", "WT300_2"}
  T14 = typedef "HEWH Calc and Calibration.ctl" = cluster{"Mean SD Var Max Min Array":string[][], "Draw Statistics (DBL)":dbl[][], "Calibration Coefficients DBL":dbl[][], "Start Gallons":dbl, "Starting Temp Decline":dbl, "K-Factor (Temperature)":dbl, "All Draw Stats":string[][], "RTD Terminate Value":dbl, "K-Factor (Flow)":dbl, "Intellifaucet Type":string, "Gas Thermal Stabilization Array":dbl[][], "Gas Thermal Stabil Complete":bool, "Gas Thermal Time":dbl, "Therm Reset Cmpt 1":bool, "Therm Reset Cmpt 2":bool, "Last Flow Rate (Therm)":dbl, "State":enum16{"State 0", "State 1", "State 2", "State 3", "State 4", "State 5", "State 6"}, "Gas Thermal Time 2":dbl}
  T15 = typedef "File Setup.lvlib/Save File DOE LabView Program.ctl" = enum16{"No Name Found", "DOE Stand", "Dishwasher Kitchen", "Portable Stand", "HEWH", "Dryer", "Dryer WILT", "HCC", "PRAT", "HEWH RLT", "Refrigeration", "Gas Water Heater"}
  T16 = typedef "Station ID Selector.ctl" = enum16{"", "A", "B", "C", "D", "Global"}
  T17 = typedef "RANGE ANSI Rate.ctl" = cluster{"Array 1":dbl[], "Array 3":dbl[], "Array 2":dbl[], "Start ANSI":bool, "ANSI Start Time":dbl, "Restart ANSI":bool, "15 Min ANSI Avg (BTU/hr)":dbl, "20 Min ANSI Avg (BTU/hr)":dbl, "25 Min ANSI Avg (BTU/hr)":dbl, "Absolute Pressure":dbl, "Gas Temperature":dbl, "Volumetric Flow Rate":dbl, "Mass Flow Rate":dbl, "Array 4":dbl[], "Array 5":dbl[], "Gas Rate":dbl, "15 Min Pres Avg (PSIA)":dbl, "20 Min Pres Avg (PSIA)":dbl, "25 Min Pres Avg (PSIA)":dbl, "15 Min Temp Avg (°F) ":dbl, "20 Min Temp Avg (°F)":dbl, "25 Min Temp Avg (°F)":dbl, "15 Min Uncorrected Avg (CFH)":dbl, "20 Min Uncorrected Avg (CFH)":dbl, "25 Min Uncorrected Avg (CFH)":dbl, "15 Min Corrected Avg (SCFH)":dbl, "20 Min Corrected Avg (SCFH)":dbl, "25 Min Corrected Avg (SCFH)":dbl, "15 Min Complete":bool, "20 Min Complete":bool, "25 Min Complete":bool, "Heating Value (BTU/ft³)":dbl}
  T18 = typedef "Data Cluster.ctl" = cluster{"Absolute Pressure":dbl, "Gauge/Diff. Pressure":dbl, "Barometric Pressure":dbl, "Temperature":dbl, "Volumetric Flow":dbl, "Mass Flow":dbl, "Setpoint":dbl, "Valve Drive":dbl, "Totalizer":dbl, "[hr]":dbl, "[min]":dbl, "[sec]":dbl, "Totalizer Average Flow":dbl, "Totalizer Peak Flow":dbl, "Gas selected":string}
  T19 = typedef "HEWH Draw Parameters.ctl" = cluster{"Draws Left":i32, "Draws Left Array":i32[], "Remaining Draws (A)":i32, "Remaining Draws (B)":i32, "Remaining Draws (C)":i32, "Remaining Draws (D)":i32, "Index of Element (A-D)":i32[], "Station A":T2, "Station B":T2, "Station C":T2, "Station D":T2}
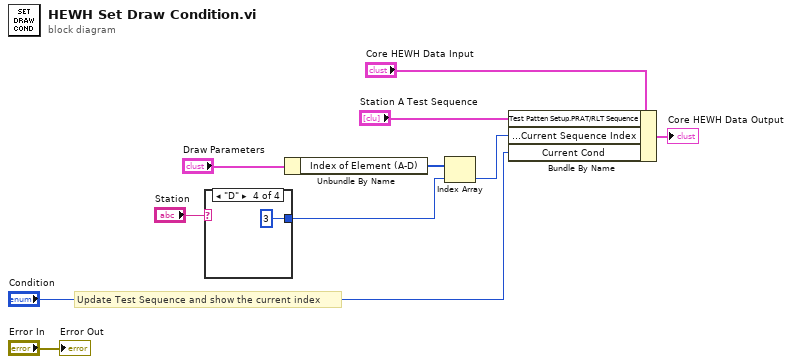
[diagram p0: block diagram]
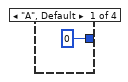
[diagram p2: hidden frame]
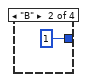
[diagram p3: hidden frame]
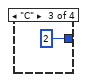
[diagram p4: hidden frame]
diagram:
  # "Update Test Sequence and show the current index"
  n1 = case shown="\"D\"" "Station" {
    tunnel: [0 ("index") 1 ("index") 2 ("index") 3 ("index")] -> w6
    frame "A", Default {
    }
    frame "B" {
    }
    frame "C" {
    }
    frame "D" {
    }
  }
  n2 = Unbundle By Name("Draw Parameters") -> ("Index of Element (A-D)"=w7:i32[])
  n3 = Index Array(array=w7, index=w6) -> (element=w5:i32)
  n4 = Bundle By Name(cluster="Core HEWH Data Input", "Test Patten Setup.PRAT/RLT Sequence"="Station A Test Sequence", "Test Patten Setup.Current Sequence Index"=w5, "Current Cond"="Condition") -> (→"Core HEWH Data Output":T8)
  "Error Out" <- "Error In"
